vi "_Parse ES Flatness Limit Check Result.vi"(8 "error in (no error)":errorcluster, 10 "Input String":string, 11 "VISA resource name":refnum<visa-resource-name>) -> (0 "error out":errorcluster, 1 "Limit Check Results":T1, 2 "Reliability":i32, 3 "VISA resource name out":refnum<visa-resource-name>, 5 "Out Of Tolerance":i32)   [LabVIEW 2020, in "Rohde&Schwarz CMWXP NR FR1 Measurement.lvlib"]
uses:
  <instrlib>/Rohde&Schwarz CMWXP NR FR1 Measurement/Rohde&Schwarz CMWXP NR FR1 Measurement.lvlib
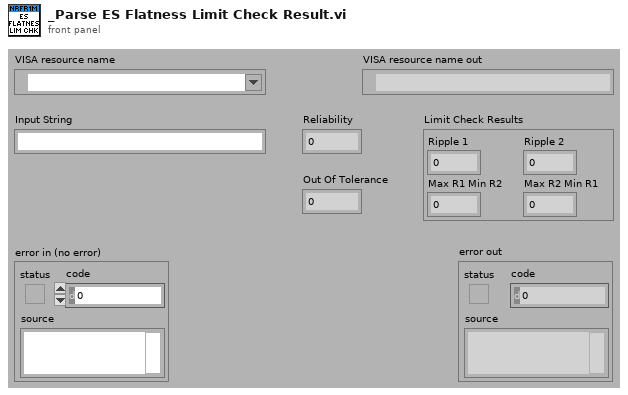
[diagram p1: front panel]
types:
  T1 = cluster{"Ripple 1":i32, "Ripple 2":i32, "Max R1 Min R2":i32, "Max R2 Min R1":i32}
  T2 = cluster{"Limit Check Value":i32, "Limit Check Value":i32, "Limit Check Value":i32, "Limit Check Value":i32}
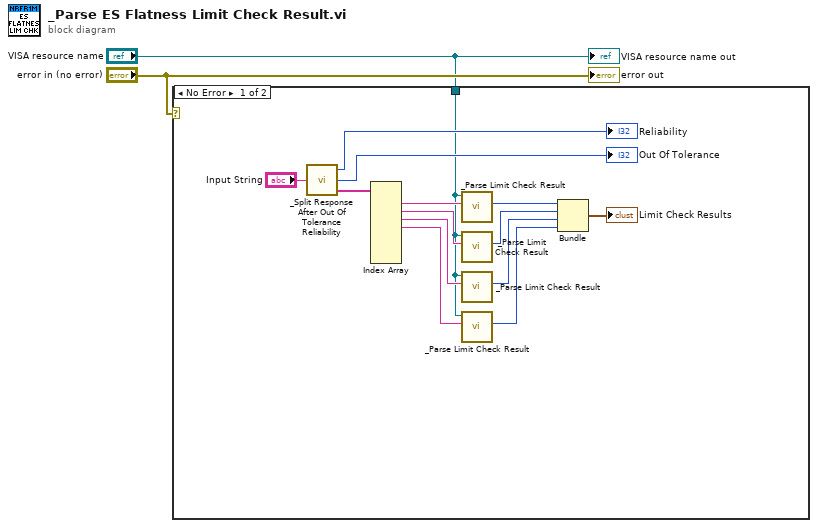
[diagram p0: block diagram]
diagram:
  n1 = case shown="No Error" "error in (no error)" {
    tunnel: "VISA resource name" -> [w4 _]
    frame No Error {
      n2 = call <instrlib>:"_Split Response After Out Of Tolerance Reliability.vi"("Input String"="Input String") -> ("Reliability out"=→"Reliability":i32, "Out Of Tolerance"=→"Out Of Tolerance":i32, "Response out"=w12:string[])
      n3 = Index Array(array=w12) -> (element #1=w11:string, element #2=w10:string, element #3=w8:string, element #4=w9:string)  [unwired: 8 in, 4 out]
      n4 = call <instrlib>:"_Parse Limit Check Result.vi"("String Value In"=w11, "VISA resource name"=w4) -> ("Limit Check Value"=w16:i32)  [unwired: 7 in, 2 out]
      n5 = call <instrlib>:"_Parse Limit Check Result.vi"("String Value In"=w10, "VISA resource name"=w4) -> ("Limit Check Value"=w15:i32)  [unwired: 7 in, 2 out]
      n6 = call <instrlib>:"_Parse Limit Check Result.vi"("String Value In"=w8, "VISA resource name"=w4) -> ("Limit Check Value"=w7:i32)  [unwired: 7 in, 2 out]
      n7 = call <instrlib>:"_Parse Limit Check Result.vi"("String Value In"=w9, "VISA resource name"=w4) -> ("Limit Check Value"=w6:i32)  [unwired: 7 in, 2 out]
      n8 = Bundle("Limit Check Value"=w16, "Limit Check Value"=w15, "Limit Check Value"=w7, "Limit Check Value"=w6) -> (→"Limit Check Results":T2)  [unwired: 1 in]
    }
    frame Error {
    }
  }
  "VISA resource name out" <- "VISA resource name"
  "error out" <- "error in (no error)"
